vi "Compute Average.vi"(8 "error in (no error)":errorcluster, 11 "Video Frame in":refnum<class "Video Frame.lvclass">) -> (0 "error out":errorcluster, 1 "Standard Deviation":dbl, 2 "Average":dbl, 3 "Video Frame out":refnum<class "Video Frame.lvclass">)   [LabVIEW 2018, in "Video Frame.lvclass"]
uses:
  Video Frame.lvclass
  Video Frame.lvclass/Video Frame.ctl
  Standard Averager/Standard Averager.lvclass
  C:/Users/aaron.jencks/Documents/GitHub/emerson_seed_object_detection/LabVIEW/Projects/Paul's Video Viewer/Classes/Averager/Averager.lvclass
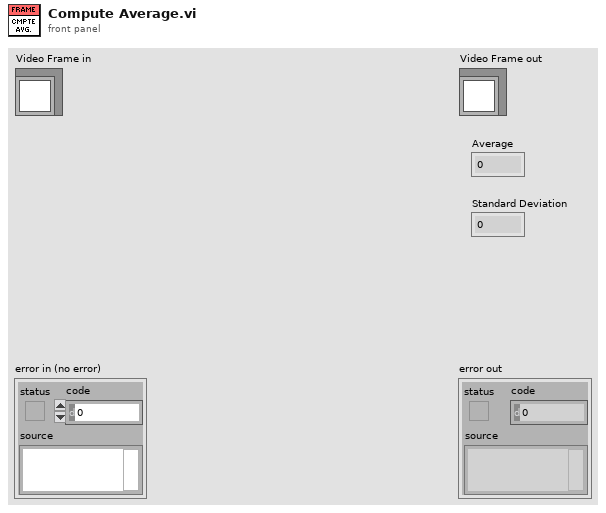
[diagram p1: front panel]
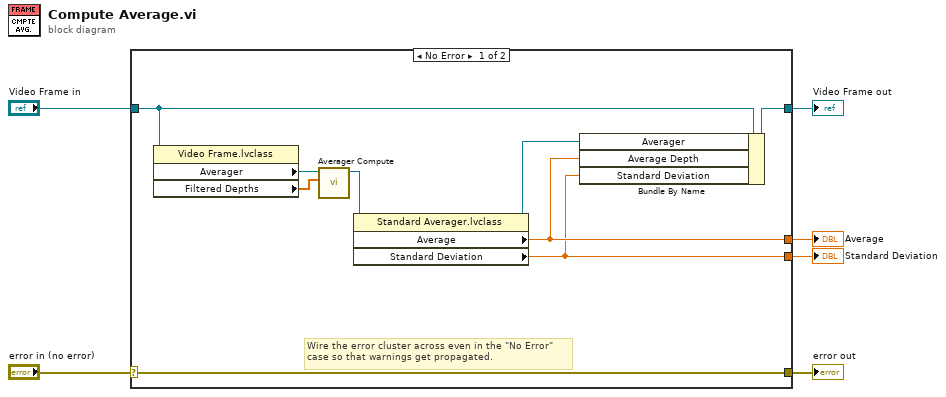
[diagram p0: block diagram]
diagram:
  n1 = case shown="No Error" "error in (no error)" {
    selector: "error in (no error)" -> [w15 w17]
    tunnel: [w15 w17] -> w5
    tunnel: [w10 w16] -> w3
    tunnel: "Video Frame in" -> [w11 w16]
    tunnel: [w8 _] -> w2
    tunnel: [w7 _] -> w1
    frame No Error {
      # "Wire the error cluster across even in the \"No Error\"\ncase so that warnings get propagated."
      n2 = property class="Video Frame.lvclass"(reference=w11) -> ("Averager"=w14:refnum<class "Standard Averager.lvclass">, "Filtered Depths"=w13:dbl[])  [unwired: 1 in, 2 out]
      n3 = call-dynamic "Averager Compute.vi"("Data"=w13, "Standard Averager in"=w14) -> ("Standard Averager out"=w12:refnum<class "Standard Averager.lvclass">)  [unwired: 8 in, 1 out]
      n4 = property class="Standard Averager.lvclass"(reference=w12) -> (reference out=w9:refnum<class "Standard Averager.lvclass">, "Average"=w8:dbl, "Standard Deviation"=w7:dbl)  [unwired: 1 in, 1 out]
      n5 = Bundle By Name(cluster=w11, "Averager"=w9, "Average Depth"=w8, "Standard Deviation"=w7) -> (w10:refnum<class "Video Frame.lvclass">)
    }
    frame Error {
    }
  }
  "error out" <- w5
  "Video Frame out" <- w3
  "Standard Deviation" <- w1
  "Average" <- w2
